vi "GeneratePieceOfSignal_TU.vi"() -> ()   [LabVIEW 2025]
uses:
  wfm-type.ctl
panel:
  out "wfm out":waveform(dbl)(graph)
  out "error out":errorcluster
  in  "wfm type":T1
  in  "frequency":dbl=1e-06 min=1e-06
  in  "amplitude":dbl
  in  "noise RMS":dbl=1.0 format="%.2p"
  in  "#s":dbl=1.0 min=1.0
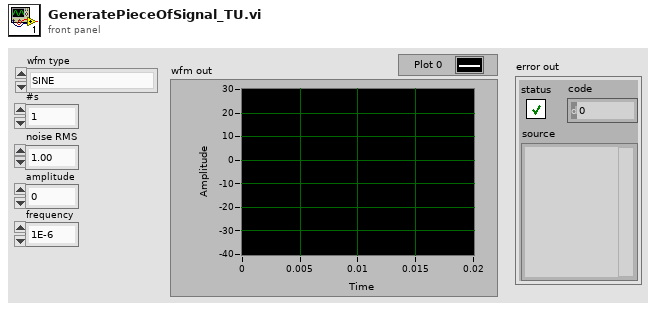
[diagram p1: front panel]
types:
  T1 = typedef "wfm-type.ctl" = enum16{"SINE", "SQUARE", "TRIANGLE", "SAWTOOTH"}
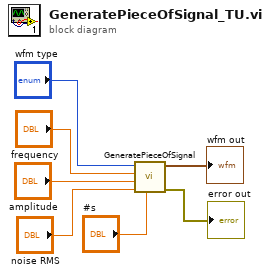
[diagram p0: block diagram]
diagram:
  n1 = call "GeneratePieceOfSignal.vi"("#s"="#s", "noise RMS"="noise RMS", "amplitude"="amplitude", "frequency"="frequency", "wfm type"="wfm type") -> ("error out"=→"error out":errorcluster, "wfm out"=→"wfm out":waveform(dbl))  [unwired: 5 in]
